vi "Write transmission data unit.vi"(8 "error in (no error)":errorcluster, 10 "Transmission Data Unit":refnum<class "Transmission Data Unit.lvclass">, 11 "Master CR in":refnum<class "Master CR.lvclass">) -> (0 "error out":errorcluster, 3 "Master CR out":refnum<class "Master CR.lvclass">)   [LabVIEW 2021]
uses:
  Master CR.lvclass
  Modbus_v121c/Transmission Data Unit/Transmission Data Unit.lvclass
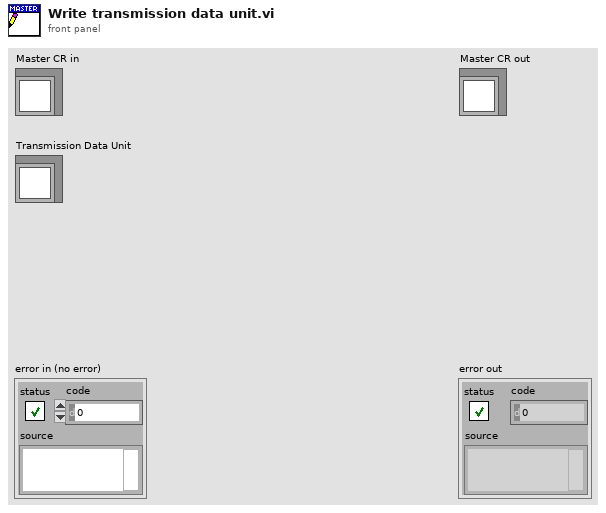
[diagram p1: front panel]
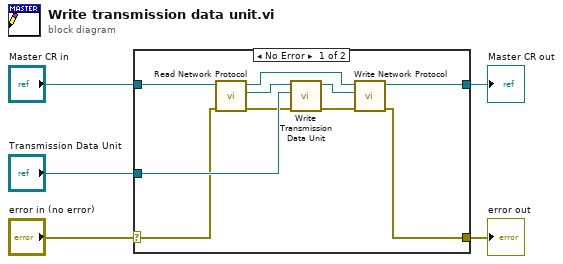
[diagram p0: block diagram]
diagram:
  n1 = case shown="No Error" "error in (no error)" {
    selector: "error in (no error)" -> [w8 w16]
    tunnel: [w7 w16] -> w4
    tunnel: [w6 w17] -> w2
    tunnel: "Master CR in" -> [w14 w17]
    tunnel: "Transmission Data Unit" -> [w15 _]
    frame No Error {
      n2 = call "Read Network Protocol.vi"("error in (no error)"=w8, "Master CR in"=w14) -> ("error out"=w10:errorcluster, "Network Protocol"=w13:refnum<class "Network Protocol.lvclass">, "Master CR out"=w11:refnum<class "Master CR.lvclass">)  [unwired: 7 in]
      n3 = call "Write Transmission Data Unit.vi"("error in (no error)"=w10, "Transmission Data Unit"=w15, "Network Protocol in"=w13) -> ("error out"=w9:errorcluster, "Network Protocol out"=w12:refnum<class "Network Protocol.lvclass">)  [unwired: 7 in]
      n4 = call "Write Network Protocol.vi"("error in (no error)"=w9, "Network Protocol"=w12, "Master CR in"=w11) -> ("error out"=w7:errorcluster, "Master CR out"=w6:refnum<class "Master CR.lvclass">)  [unwired: 7 in]
    }
    frame Error {
    }
  }
  "error out" <- w4
  "Master CR out" <- w2
